vi "test_ccd_all.vi"() -> ()   [LabVIEW 2023]
uses:
  30205172-ae8d-4653-b132-e29d8f7b38e6.vi
panel:
  out "error out":errorcluster
  in  "error in":errorcluster
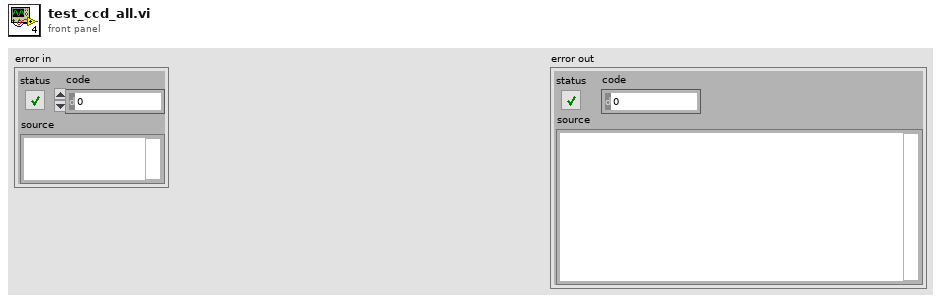
[diagram p1: front panel]
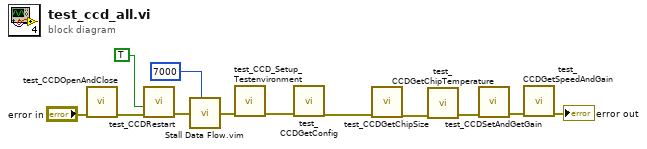
[diagram p0: block diagram]
diagram:
  n1 = call "test_CCDOpenAndClose.vi"("error in"="error in") -> ("error out"=w12:errorcluster)  [unwired: 10 in]
  n2 = call "test_CCDRestart.vi"("error in"=w12, "tear down connection"=TRUE) -> ("error out"=w10:errorcluster)  [unwired: 9 in]
  n3 = call "Stall Data Flow.vim"("value in"=w10, "milliseconds to wait"=u32 7000) -> ("value out"=w4:errorcluster)  [unwired: 1 out]
  n4 = call "test_CCD_Setup_Testenvironment.vi"("error in"=w4) -> ("error out"=w3:errorcluster)  [unwired: 7 in, 3 out]
  n5 = call "test_CCDGetConfig.vi"("error in"=w3) -> ("error out"=w8:errorcluster)  [unwired: 10 in]
  n6 = call "test_CCDGetChipSize.vi"("error in"=w8) -> ("error out"=w7:errorcluster)  [unwired: 10 in]
  n7 = call "test_CCDGetChipTemperature.vi"("error in"=w7) -> ("error out"=w6:errorcluster)  [unwired: 10 in]
  n8 = call "test_CCDSetAndGetGain.vi"("error in"=w6) -> ("error out"=w5:errorcluster)  [unwired: 10 in]
  n9 = call "test_CCDGetSpeedAndGain.vi"("error in"=w5) -> ("error out"=→"error out":errorcluster)  [unwired: 8 in, 2 out]
